vi "Get Range.vi"(8 "Error In":errorcluster, 11 "Graph In":refnum<class "Graph.lvclass">) -> (0 "Error Out":errorcluster, 2 "Range":T1, 3 "Graph Out":refnum<class "Graph.lvclass">)   [LabVIEW 2019, in "Graph.lvclass"]
uses:
  Graph.lvclass
  Public/Controls/Range.ctl
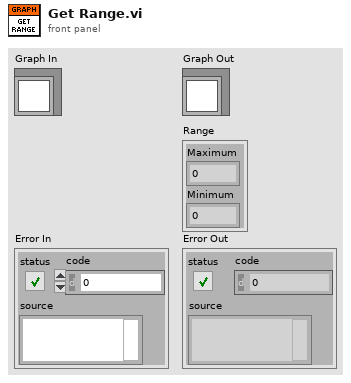
[diagram p1: front panel]
types:
  T1 = typedef "Graph.lvclass/Range.ctl" = cluster{"Maximum":i32, "Minimum":i32}
  T2 = typedef "Graph.lvclass/Data.ctl" = cluster{"Height":u32, "Width":u32, "Range":T1, "Data":i32[], "Fill To":T3}
  T3 = typedef "Graph.lvclass/Fill To.ctl" = enum16{"None", "Zero", "Inf", "-Inf"}
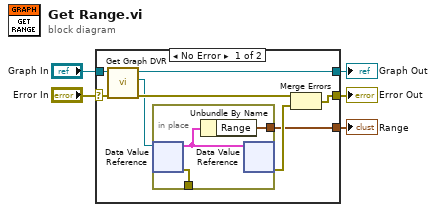
[diagram p0: block diagram]
diagram:
  n1 = case shown="No Error" "Error In" {
    selector: "Error In" -> [w9 w17]
    tunnel: [w11 w17] -> w3
    tunnel: [w6 w18] -> w4
    tunnel: "Graph In" -> [w10 w18]
    tunnel: [w12 _] -> w1
    frame No Error {
      n2 = call "Get Graph DVR.vi"("Error In"=w9, "Graph In"=w10) -> ("Error Out"=w8:errorcluster, "DVR"=w7:refnum<data-value>, "Graph Out"=w6:refnum<class "Graph.lvclass">)  [unwired: 7 in]
      n3 = in-place {
        in-place-border: [w14] -> w12
        in-place-border: [w16] -> _
        n4 = in-place-dvr #1(w7) -> (w15:T2, w16:errorcluster)
        n5 = Unbundle By Name(w15) -> ("Range"=w14:T1)
        n6 = in-place-dvr #1(w15) -> (w13:errorcluster)  [unwired: 1 out]
      }
      n7 = Merge Errors(w8, w13) -> (w11:errorcluster)
    }
    frame Error {
    }
  }
  "Graph Out" <- w4
  "Error Out" <- w3
  "Range" <- w1
